vi "Read_SR830_buffer.vi"() -> ()   [LabVIEW 2014]
panel:
  in  "error in (no error)":errorcluster
  out "error out":errorcluster
  out "String 4":string
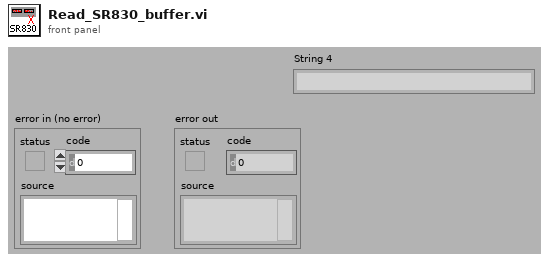
[diagram p1: front panel]
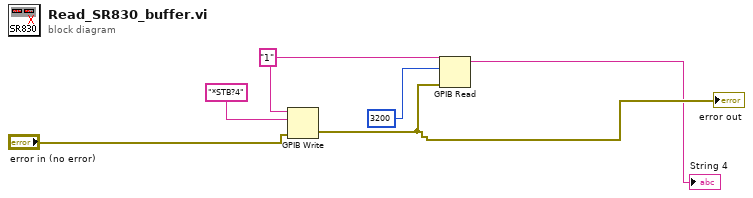
[diagram p0: block diagram]
diagram:
  w2 = "1"
  n1 = GPIB Write(0:w2, 1:"*STB?4", 3:"error in (no error)") -> (6:w4:errorcluster)  [unwired: 2 in, 1 out]
  "error out" <- w4
  n2 = GPIB Read(0:w2, 1:3200, 3:w4) -> (5:→"String 4":string)  [unwired: 2 in, 2 out]
